vi "ConfFileParser.vi"(0 "TEXT":string, 1 "search string":string) -> (2 "Cluster Array":T1(array[cluster]), 3 "Names":string[](array[string]), 4 "Codes":string[](array[string]))   [LabVIEW 2009]
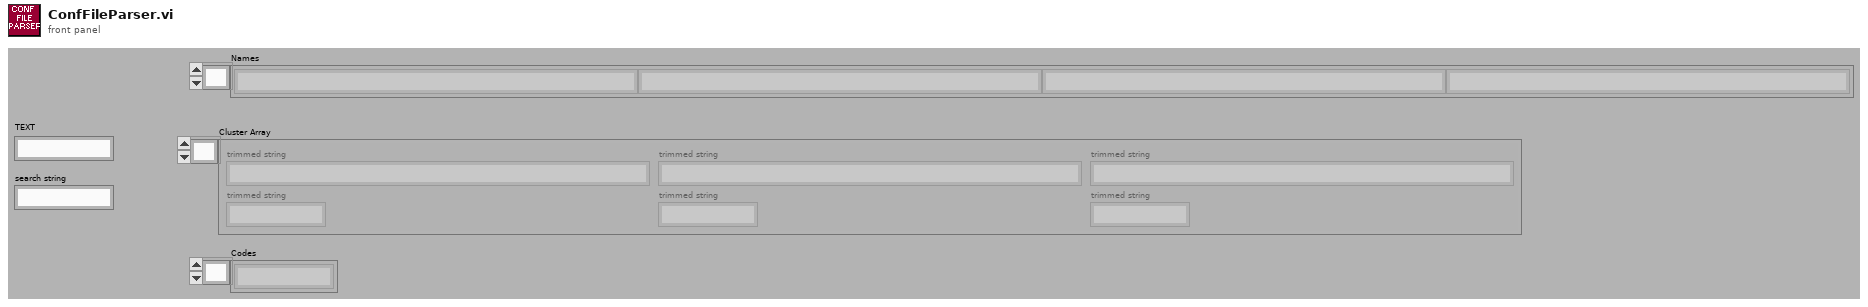
[diagram p1: front panel]
types:
  T1 = cluster{"trimmed string":string, "trimmed string":string}[]
  T2 = cluster{"trimmed string":string, "trimmed string":string}
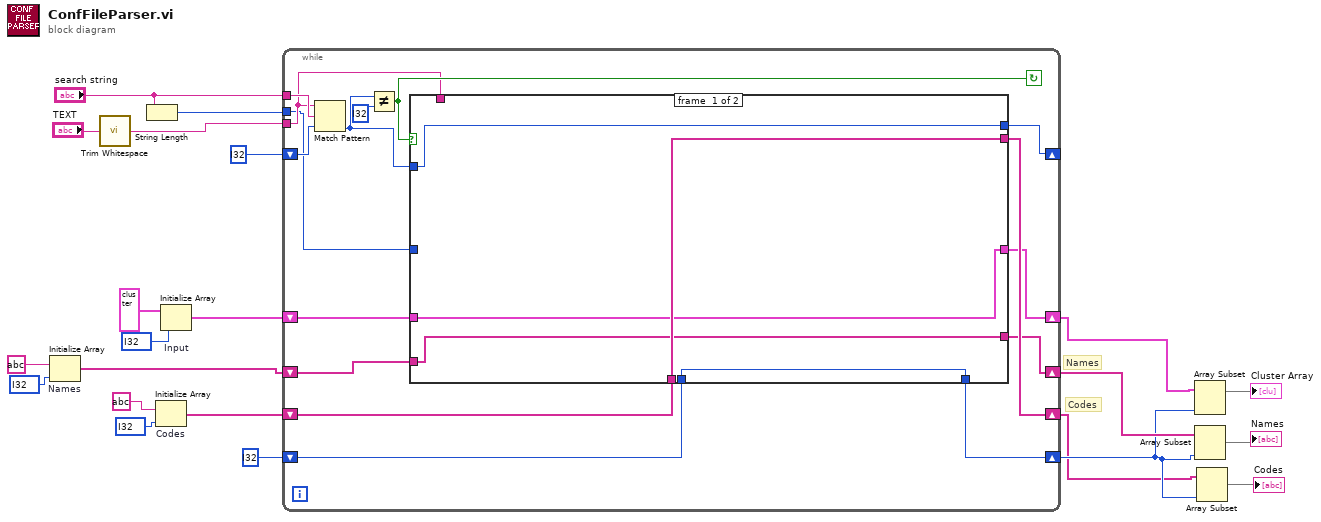
[diagram p0: block diagram]
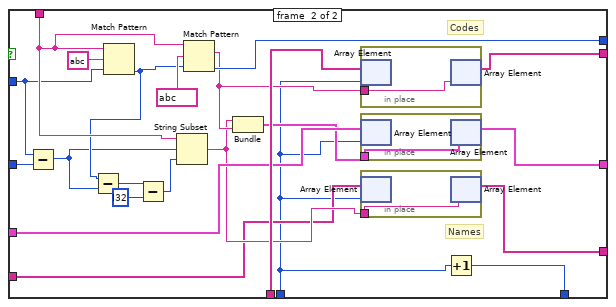
[diagram p2: hidden frame]
diagram:
  # "Names"
  # "Codes"
  n1 = Initialize Array "Names"(string ? ("trimmed string"), i32 ? ("dimension size")) -> (w14:string[])
  n2 = call <vilib>:"Trim Whitespace.vi"("string"="TEXT") -> ("trimmed string"=w13:string)  [unwired: 1 in]
  n3 = String Length(string="search string") -> (length=w9:i32)
  n4 = Initialize Array "Codes"(string ? ("trimmed string"), i32 ? ("dimension size")) -> (w11:string[])
  n5 = Initialize Array "Input"(T2 ? ("output cluster"), i32 ? ("dimension size")) -> (w15:T1)
  n6 = while {
    tunnel: "search string" -> [w36]
    tunnel: w13 -> [w34]
    shift-right: [w29] -> _
    shift-left: i32 ? ("offset (0)") -> [w31]
    shift-right: [w26] -> w7
    shift-left: w15 -> [w27]
    shift-right: [w23] -> w5
    shift-left: w14 -> [w25]
    shift-right: [w32] -> w1
    shift-left: w11 -> [w33]
    tunnel: w9 -> [w30]
    shift-right: [w24] -> w3
    shift-left: i32 ? ("dimension size") -> [w28]
    stop <- w37 continue-if-true
    n7 = Match Pattern(string=w34, regular expression=w36, offset (0)=w31) -> (offset past match=w35:i32)  [unwired: 3 out]
    n8 = Not Equal?(x=w35, y=i32 ?) -> (x != y?=w37:bool)
    n9 = case shown="True" w37 {
      tunnel: w34 -> [_ w63]
      tunnel: w35 -> [w42 w62]
      tunnel: w33 -> [w43 w53]
      tunnel: [w43 w51] -> w32
      tunnel: w30 -> [_ w58]
      tunnel: [w42 w60] -> w29
      tunnel: w28 -> [w41 w44]
      tunnel: w27 -> [w40 w50]
      tunnel: [w40 w49] -> w26
      tunnel: w25 -> [w39 w45]
      tunnel: [w41 w59] -> w24
      tunnel: [w39 w46] -> w23
      frame #0 {
      }
      frame #1 {
        # "Names"
        # "Codes"
        n10 = Subtract(x=w62, y=w58) -> (x-y=w57:i32)
        n11 = Match Pattern(string=w63, regular expression=string ? ("search string"), offset (0)=w62) -> (offset past match=w61:i32)  [unwired: 3 out]
        n12 = Subtract(x=w61, y=w57) -> (x-y=w55:i32)
        n13 = Subtract(x=w55, y=i32 ?) -> (x-y=w54:i32)
        n14 = String Subset(string=w63, offset (0)=w57, length (rest)=w54) -> (substring=w47:string)
        n15 = Match Pattern(string=w63, regular expression=string ?, offset (0)=w61) -> (match substring=w52:string, offset past match=w60:i32)  [unwired: 2 out]
        n16 = Bundle("trimmed string"=w47, "trimmed string"=w52) -> (w48:T2)  [unwired: 1 in]
        n17 = in-place {
          in-place-border: w52 -> [w68]
          n18 = in-place-array #1(w53, w44) -> ()  [unwired: 1 out]
          n19 = in-place-array #1(w68) -> (w51:string[])  [unwired: 1 out]
        }
        n20 = in-place {
          in-place-border: w48 -> [w67]
          n21 = in-place-array #2(w50, w44) -> ()  [unwired: 1 out]
          n22 = in-place-array #2(w67) -> (w49:T1)  [unwired: 1 out]
        }
        n23 = in-place {
          in-place-border: w47 -> [w66]
          n24 = in-place-array #3(w45, w44) -> ()  [unwired: 1 out]
          n25 = in-place-array #3(w66) -> (w46:string[])  [unwired: 1 out]
        }
        n26 = Increment(x=w44) -> (x+1=w59:i32)
      }
    }
  }
  n27 = Array Subset(array=w7, length=w3) -> (→"Cluster Array":T1)  [unwired: 1 in]
  n28 = Array Subset(array=w5, length=w3) -> (→"Names":string[])  [unwired: 1 in]
  n29 = Array Subset(array=w1, length=w3) -> (→"Codes":string[])  [unwired: 1 in]
